vi "About.vi"() -> ()   [LabVIEW 2015]
panel:
  in  "OK Button":bool
  # "Справка:\nДананя демка демонстириует использование TelegramBotAPI в LabVIEW. С помощью \nсообщений в месенджере Telegram, можно изменять характер свечения пользовательских \nсветодиодов LED1-3  на myRIO 1900 и выполнять некоторые другие функции.\n\nДля корректной работы:\n1. Необходимо создать бота [1] в Telegram и вписать в поле \"Token\" токен, выданный @Botfather [2].\n2. На своём устройстве создать личный чат с созданным на предыдущем шаге ботом.\n2.1 Для тестирования можно использовать бота @ATISIndBoT\n\nДля изменения характера свчения LED:\n3.1 Отправлять в чат сообщения формата \"/led#,Period(ms/us),DutyCycle(%)\", например /led1,1000,50. \nДля  LED1,2 период задаётся в ms, для LED3 в us.  Изменение характера свечения осуществляется \nпосредстам PWM.\n3.2 Отправлять в чат сообщения формата \"/led#\" без параметров. Бот вернёт пользовательскую \nклавиатуру с несколькими кнопками, позволяющими зажигать/тушить светодиод.\n\nДля получения текущего времени myRIO:\n3.3 Отправить в чат команду \"/gettime\"\n\nДля получения данных о погоде в определённом городе:\n3.4 Отправить команду \"/getweather,Сity,Region\", city - обязательный параметр, region - необязательеный параметр.\nНапример, чтобы получить данные о погоде в городе Астана (Казахстан) необходимо передать боту \nкоманду: /getweather,astana,kz\n                                                                                                                                                                              \nИсточники:\n1. https://core.telegram.org/bots#6-botfather\n2. https://core.telegram.org/bots/api#authorizing-your-bot\n                                                                                                                                                    Обратная связь: vadimladik@gmail.com"
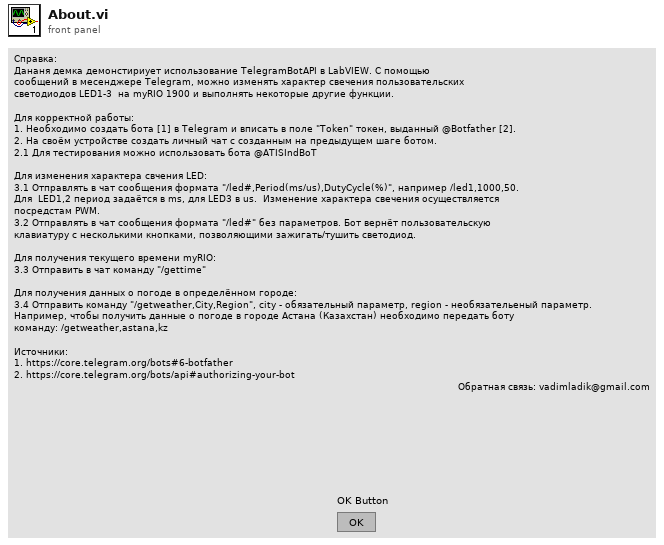
[diagram p1: front panel]
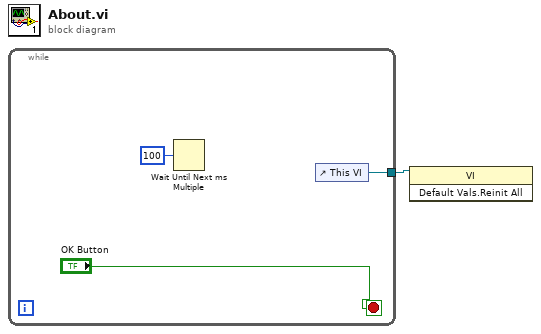
[diagram p0: block diagram]
diagram:
  n1 = while {
    tunnel: [w3] -> w1
    stop <- "OK Button" stop-if-true
    n2 = Wait Until Next ms Multiple(millisecond multiple=u32 100) -> ()  [unwired: 1 out]
    n3 = control-ref of="This VI"() -> (w3:refnum<vi>)
  }
  n4 = invoke class="VI" method="Default Vals.Reinit All"(reference=w1) -> ()  [unwired: 2 in, 3 out]
